vi "Close.vi"(8 "error in (no error)":errorcluster, 11 "SQLite Connection in":refnum<class "Connection.lvclass">) -> (0 "error out":errorcluster)   [LabVIEW 2013, in "SQLiteSupport.lvlib" / "Connection.lvclass"]
doc: "Closes the connection to the SQLite3 database file."
uses:
  Connection.lvclass
  Connection.lvclass/Connection.ctl
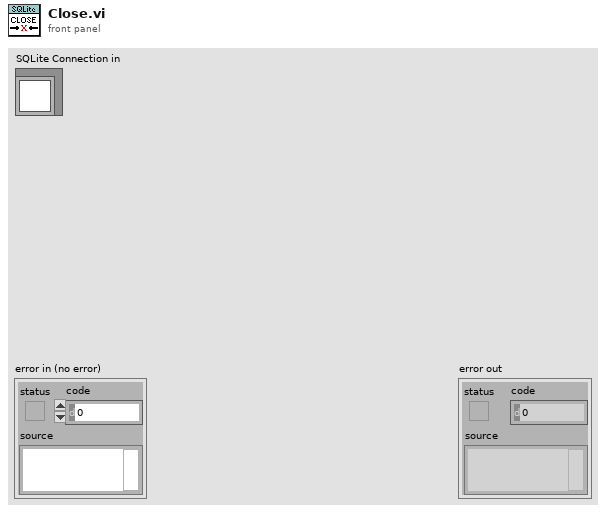
[diagram p1: front panel]
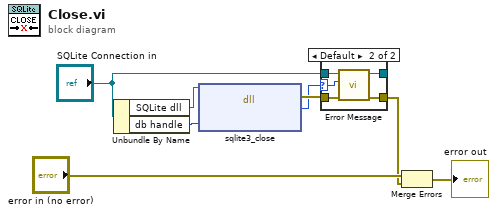
[diagram p0: block diagram]
diagram:
  n1 = Unbundle By Name("SQLite Connection in") -> ("SQLite dll"=w5:path, "db handle"=w8:u64)
  n2 = dll-call lib="C:/SQLite/sqlite3.dll" fn="sqlite3_close"(path in=w5, "handle"=w8) -> (error out=w4:errorcluster, "return code"=w3:i32)  [unwired: 3 in, 1 out]
  n3 = case shown="Default" w3 {
    selector: w3 -> [_ w11]
    tunnel: "SQLite Connection in" -> [w10 w15]
    tunnel: [w10 w14] -> _
    tunnel: w4 -> [w9 w13]
    tunnel: [w9 w12] -> w1
    frame 0 {
      # "No Error"
    }
    frame Default {
      n4 = call "Error Message.vi"("error in (no error)"=w13, "error code"=w11, "Connection in"=w15) -> ("error out"=w12:errorcluster, "Connection out"=w14:refnum<class "Connection.lvclass">)  [unwired: 7 in]
    }
  }
  n5 = Merge Errors("error in (no error)", w1) -> (→"error out":errorcluster)
